vi "Send Inline Buffer.vi"(8 "error in (no error)":errorcluster, 9 "size":u64, 10 "address":u64, 11 "Plugin Interface in":refnum<class "Plugin Interface.lvclass">) -> (0 "error out":errorcluster, 3 "Plugin Interface out":refnum<class "Plugin Interface.lvclass">)   [LabVIEW 2017, in "DSF Core.lvlib" / "Plugin Interface.lvclass"]
uses:
  Plugin Interface.lvclass
  C:/Git/DSF/Data Sharing Framework/Source/Core/Engine/Classes/Interfaces/Interface/Interface.lvclass
  Command Data.ctl
  Command.ctl
  Command Parameters.ctl
  Interface/Interface.lvclass/Interface.ctl
  Response.ctl
  Send Plugin Command.vi
  Interface/Send Command.vi
  Interface/Write RT FIFO.vi
  Dispatcher/Command Timeout.vi
  Wait For Plugin Response.vi
  Dispatcher/Invalid Response Parameters.vi
  Dispatcher/Invalid Response.vi
  Interface/Interface.lvclass
  DSF Core.lvlib
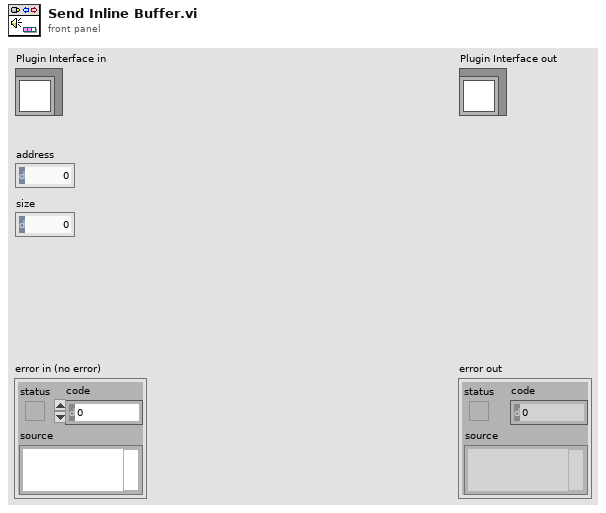
[diagram p1: front panel]
types:
  T1 = typedef "DSF Core.lvlib/Plugin Interface.lvclass/Command.ctl" = enum8{"Set Inline Buffer", "Rx", "Tx", "Shutdown"}
  T2 = typedef "DSF Core.lvlib/Plugin Interface.lvclass/Command Parameters.ctl" = cluster{"arg1":u64, "arg2":u64}
  T3 = typedef "DSF Core.lvlib/Plugin Interface.lvclass/Command Data.ctl" = cluster{"Command":T1, "Parameters":T2}
  T4 = typedef "DSF Core.lvlib/Plugin Interface.lvclass/Response Data.ctl" = cluster{"Response":T5, "Parameters":T6}
  T5 = typedef "DSF Core.lvlib/Plugin Interface.lvclass/Response.ctl" = enum8{"General Ack", "Shutting Down"}
  T6 = typedef "DSF Core.lvlib/Plugin Interface.lvclass/Response Parameters.ctl" = cluster{"arg1":u64, "arg2":u64}
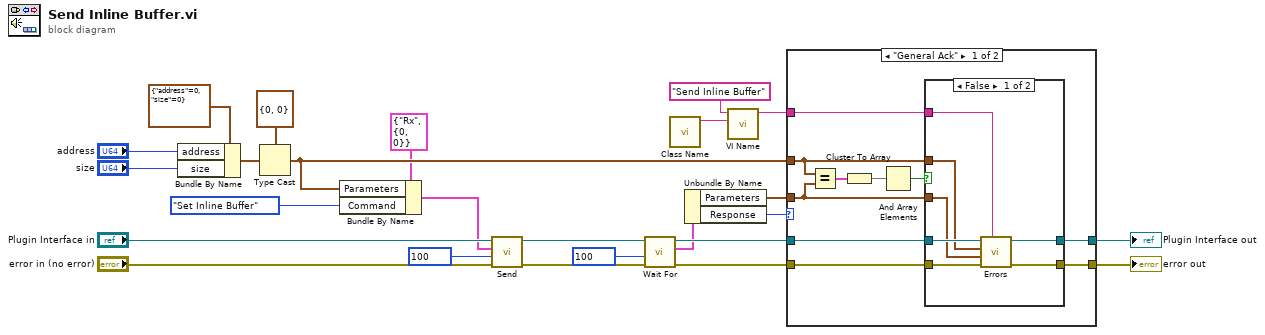
[diagram p0: block diagram]
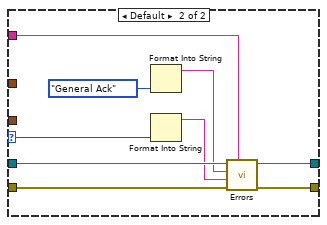
[diagram p3: hidden frame]
diagram:
  n1 = Bundle By Name(cluster=cluster{"address":u64, "size":u64} {"address"=0, "size"=0}, "address"="address", "size"="size") -> (w23:cluster{"address":u64, "size":u64})
  n2 = Type Cast(type=T2 {"arg1"=0, "arg2"=0} ("Command Parameters"), x=w23) -> (*(type *) &x=w5:T2)
  n3 = Bundle By Name(cluster=T3 {"Command"=enum."Rx", "Parameters"={"arg1"=0, "arg2"=0}} ("command"), "Parameters"=w5, "Command"=Command."Set Inline Buffer") -> (w16:T3)
  n4 = call-poly "Send.vi"("error in (no error)"="error in (no error)", "timeout in ms (0)"=100, "command"=w16, "Plugin Interface in"="Plugin Interface in") -> ("error out"=w14:errorcluster, "Plugin Interface out"=w15:refnum<class "Plugin Interface.lvclass">)  [unwired: 6 in]
  n5 = call-poly "Wait For.vi"("error in (no error)"=w14, "timeout in ms (0)"=100, "Plugin Interface in"=w15) -> ("error out"=w10:errorcluster, "response"=w8:T4, "Plugin Interface out"=w12:refnum<class "Plugin Interface.lvclass">)  [unwired: 5 in, 1 out]
  n6 = call "Class Name.vi"() -> ("class name"=w3:string)  [unwired: 11 in]
  n7 = Unbundle By Name(w8) -> ("Parameters"=w6:T6, "Response"=w7:T5)
  n8 = call "VI Name.vi"("class name (\"\")"=w3, "vi name"="Send Inline Buffer" ("error source vi name")) -> ("full VI name"=w1:string)  [unwired: 9 in]
  n9 = case shown="\"General Ack\"" w7 {
    selector: w7 -> [_ w49]
    tunnel: w12 -> [w35 w53]
    tunnel: [w33 w51] -> w11
    tunnel: w10 -> [w34 w52]
    tunnel: [w32 w50] -> w9
    tunnel: w6 -> [w27 _]
    tunnel: w5 -> [w28 _]
    tunnel: w1 -> [w26 w45]
    frame "General Ack" {
      n10 = Equal?(x=w28, y=w27) -> (x = y?=w31:cluster{"arg1":bool, "arg2":bool})
      n11 = Cluster To Array(cluster=w31) -> (array=w30:bool[])
      n12 = And Array Elements(Boolean array=w30) -> (logical AND=w29:bool)
      n13 = case shown="False" w29 {
        tunnel: w35 -> [w40 w44]
        tunnel: w34 -> [w42 w43]
        tunnel: [w39 w44] -> w33
        tunnel: [w41 w43] -> w32
        tunnel: w28 -> [w37 _]
        tunnel: w27 -> [w38 _]
        tunnel: w26 -> [w36 _]
        frame False {
          n14 = call-poly "Errors.vi"("error source vi name"=w36, "error in (no error)"=w42, "actual parameters"=w38, "expected parameters"=w37, "Interface in"=w40) -> ("error out"=w41:errorcluster, "Interface out"=w39:refnum<class "Plugin Interface.lvclass">)  [unwired: 5 in]
        }
        frame True {
          # "correct parameters"
        }
      }
    }
    frame Default {
      n15 = Format Into String(Response."General Ack" ("Response")) -> (resulting string=w46:string)  [unwired: 3 in, 1 out]
      n16 = Format Into String(w49) -> (resulting string=w48:string)  [unwired: 3 in, 1 out]
      n17 = call-poly "Errors.vi"("error source vi name"=w45, "error in (no error)"=w52, "actual response"=w48, "expected response"=w46, "Interface in"=w53) -> ("error out"=w50:errorcluster, "Interface out"=w51:refnum<class "Plugin Interface.lvclass">)  [unwired: 5 in]
    }
  }
  "error out" <- w9
  "Plugin Interface out" <- w11
